vi "Test Assert Not In Range.vi"(8 "error in (no error)":errorcluster) -> (0 "error out":errorcluster)   [LabVIEW 2013]
uses:
  classes/Test/Test.lvclass
  classes/Assert/Assert.lvclass
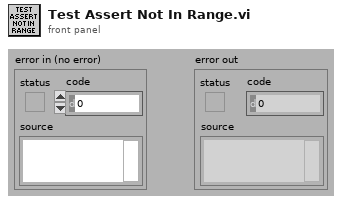
[diagram p1: front panel]
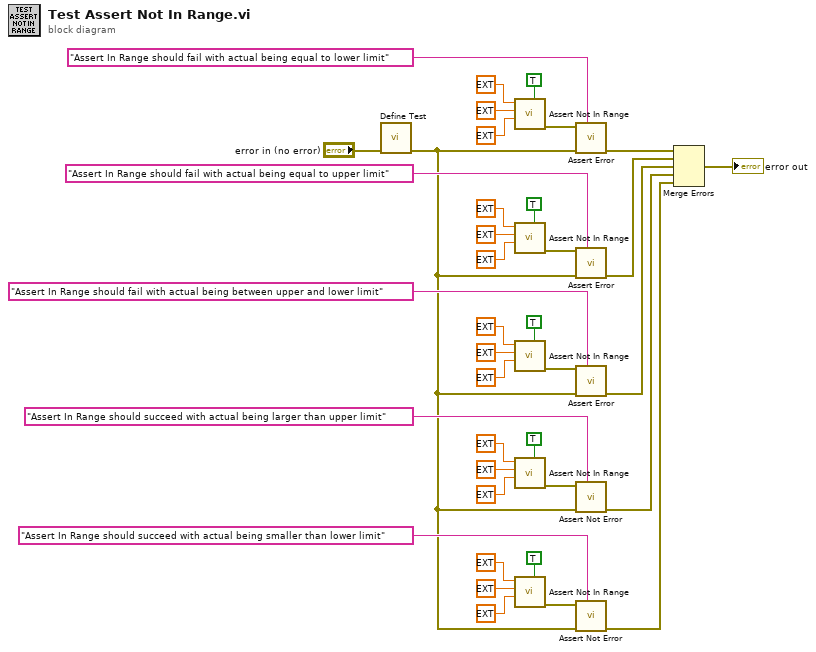
[diagram p0: block diagram]
diagram:
  n1 = call "Define Test.vi"("error in (no error)"="error in (no error)") -> ("error out"=w24:errorcluster)  [unwired: 9 in, 1 out]
  n2 = call "Assert Not In Range.vi"("Assert Only? (F)"=TRUE, "Lower Limit"=ext 7.0, "Upper Limit"=ext 10.0, "X"=ext 7.0 ("Actual")) -> ("error out"=w38:errorcluster)  [unwired: 6 in, 1 out]
  n3 = call "Assert Not In Range.vi"("Assert Only? (F)"=TRUE, "Lower Limit"=ext 7.0, "Upper Limit"=ext 10.0, "X"=ext 10.0 ("Actual")) -> ("error out"=w16:errorcluster)  [unwired: 6 in, 1 out]
  n4 = call "Assert Not In Range.vi"("Assert Only? (F)"=TRUE, "Lower Limit"=ext 7.0, "Upper Limit"=ext 10.0, "X"=ext 8.0 ("Actual")) -> ("error out"=w3:errorcluster)  [unwired: 6 in, 1 out]
  n5 = call "Assert Not In Range.vi"("Assert Only? (F)"=TRUE, "Lower Limit"=ext 7.0, "Upper Limit"=ext 10.0, "X"=ext 11.0 ("Actual")) -> ("error out"=w2:errorcluster)  [unwired: 6 in, 1 out]
  n6 = call "Assert Not In Range.vi"("Assert Only? (F)"=TRUE, "Lower Limit"=ext 7.0, "Upper Limit"=ext 10.0, "X"=ext 6.0 ("Actual")) -> ("error out"=w1:errorcluster)  [unwired: 6 in, 1 out]
  n7 = call "Assert Error.vi"("Label"="Assert In Range should fail with actual being equal to lower limit", "error in (no error)"=w24, "Error?"=w38) -> ("error out"=w32:errorcluster)  [unwired: 7 in, 1 out]
  n8 = call "Assert Error.vi"("Label"="Assert In Range should fail with actual being equal to upper limit", "error in (no error)"=w24, "Error?"=w16) -> ("error out"=w33:errorcluster)  [unwired: 7 in, 1 out]
  n9 = call "Assert Error.vi"("Label"="Assert In Range should fail with actual being between upper and lower limit", "error in (no error)"=w24, "Error?"=w3) -> ("error out"=w29:errorcluster)  [unwired: 7 in, 1 out]
  n10 = call "Assert Not Error.vi"("Label"="Assert In Range should succeed with actual being larger than upper limit", "error in (no error)"=w24, "Not Error?"=w2) -> ("error out"=w28:errorcluster)  [unwired: 7 in, 1 out]
  n11 = call "Assert Not Error.vi"("Label"="Assert In Range should succeed with actual being smaller than lower limit", "error in (no error)"=w24, "Not Error?"=w1) -> ("error out"=w25:errorcluster)  [unwired: 7 in, 1 out]
  n12 = Merge Errors(w32, w33, w29, w28, w25) -> (→"error out":errorcluster)
